vi "Vision Processing.vi"(4 "error in (no error)":errorcluster) -> ()   [LabVIEW 2019]
doc: "This VI runs in parallel to other tasks. It gets images from the camera, processes them for color or shape and uses commands or globals to affect the behavior of other subsystems."
uses:
  Framework/Robot Global Data.vi
  <vilib>/vision/NI_Vision_Development_Module.lvlib
panel:
  out "Results 2":T1(array[cluster]) {"Normalized Center"."x" format="%#_2g"; "Normalized Center"."y" format="%#_2g"; "Overall Score" format="%#_2g"; "Distance (ft)" format="%#_3g"; "Area Score" format="%#_2g"; "Moment Score" format="%#_2g"; "Aspect Score" format="%#_2g"}
  in  "Color Mode":u16(ring)=2 items=["RGB", "HSL", "HSV", "HSI"]
  out "Qualified 2":i32
  in  "LED Color Range":T2={"Hue"={92.46666717529297, 124.46666717529297}, "Sat"={154.82142857142856, 255.0}, "Val"={100.17857142857144, 251.32874298095703}} {"Hue" scale=0.0..255.0 scale format="%#_3g"}
  out "Results":T1(array[cluster]) {"Normalized Center"."x" format="%#_2g"; "Normalized Center"."y" format="%#_2g"; "Overall Score" format="%#_2g"; "Distance (ft)" format="%#_3g"; "Area Score" format="%#_2g"; "Moment Score" format="%#_2g"; "Aspect Score" format="%#_2g"}
  in  "Size Limit %":dbl=0.1 min=0.0 max=100.0 step=0.01 format="%#_13g"
  in  "Particle Count LImit":i32=5
  out "Qualified":i32
  out "Mask":T3(plugin-control)
  out "Original Image":T3(plugin-control)
  # "Scores"
  # "Scores"
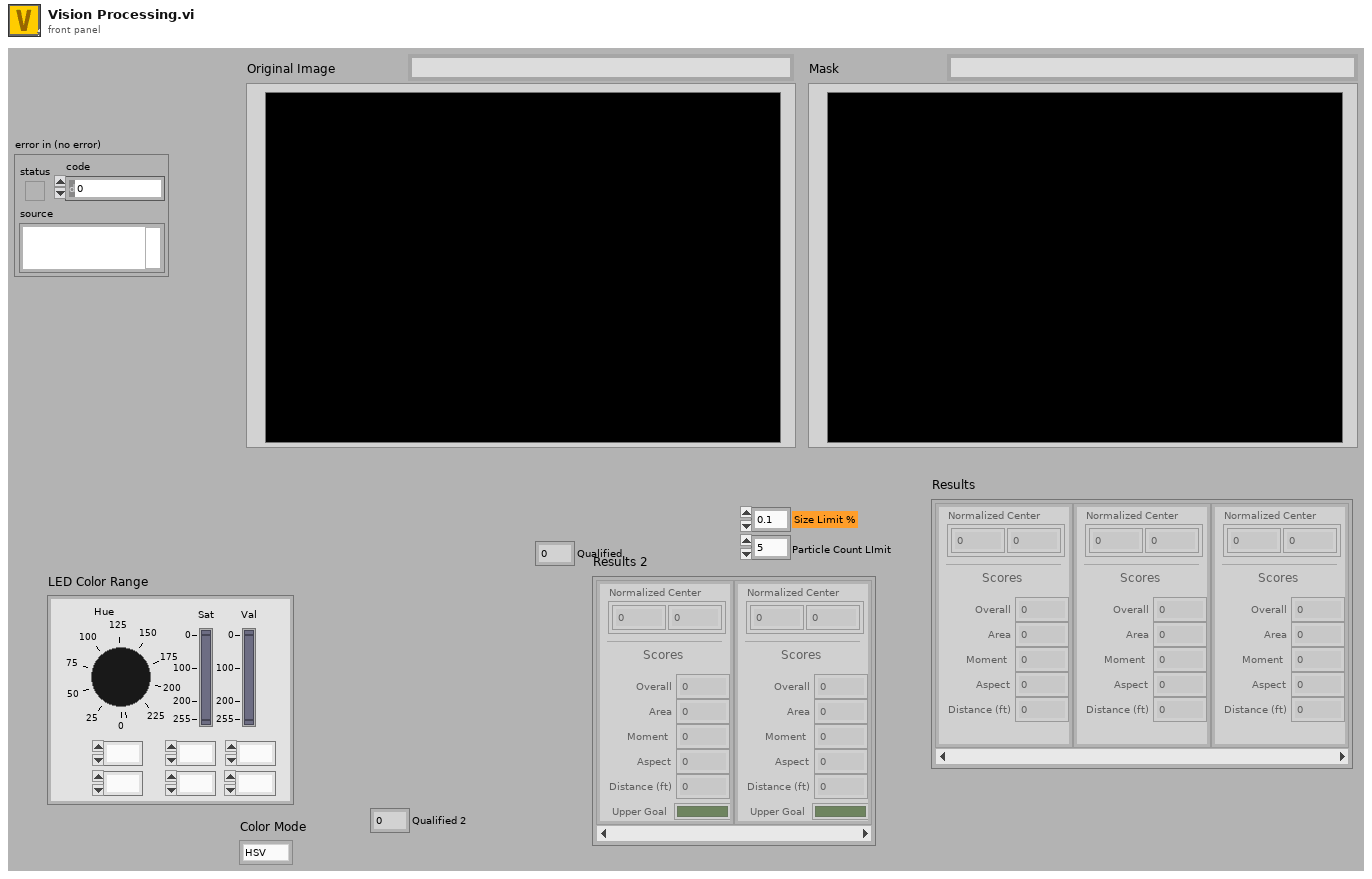
[diagram p1: front panel]
types:
  T1 = cluster{"diameter points":cluster{"first point":cluster{"x":dbl, "y":dbl}, "projected point":cluster{"x":dbl, "y":dbl}}, "Normalized Center":cluster{"x":dbl, "y":dbl}, "Overall Score":dbl, "Area Score":dbl, "Moment Score":dbl, "Aspect Score":dbl, "Distance (ft)":dbl, "Upper Goal":bool}[]
  T2 = cluster{"Hue":cluster{dbl, dbl}, "Sat":cluster{dbl, dbl}, "Val":cluster{dbl, dbl}}
  T3 = typedef "IMAQ Image.ctl" = refnum<image>
  T4 = typedef "Particle Parameters" = i32
  T5 = enum16{"Vision Off", "Ball Vision", "Feeder Station"}
  T6 = enum32{"AutoM", "Close", "Dilate", "Erode", "Gradient", "Gradient out", "Gradient in", "Hit miss", "Open", "PClose", "POpen", "Thick", "Thin"}
  T7 = typedef "Target Fields.ctl" = cluster{"diameter points":cluster{"first point":cluster{"x":dbl, "y":dbl}, "projected point":cluster{"x":dbl, "y":dbl}}, "normalized center":cluster{"x":dbl, "y":dbl}, "Overall Score":dbl, "Area Score":dbl, "Moment Score":dbl, "Aspect Score":dbl, "Distance (ft)":dbl, "Upper Goal":bool}
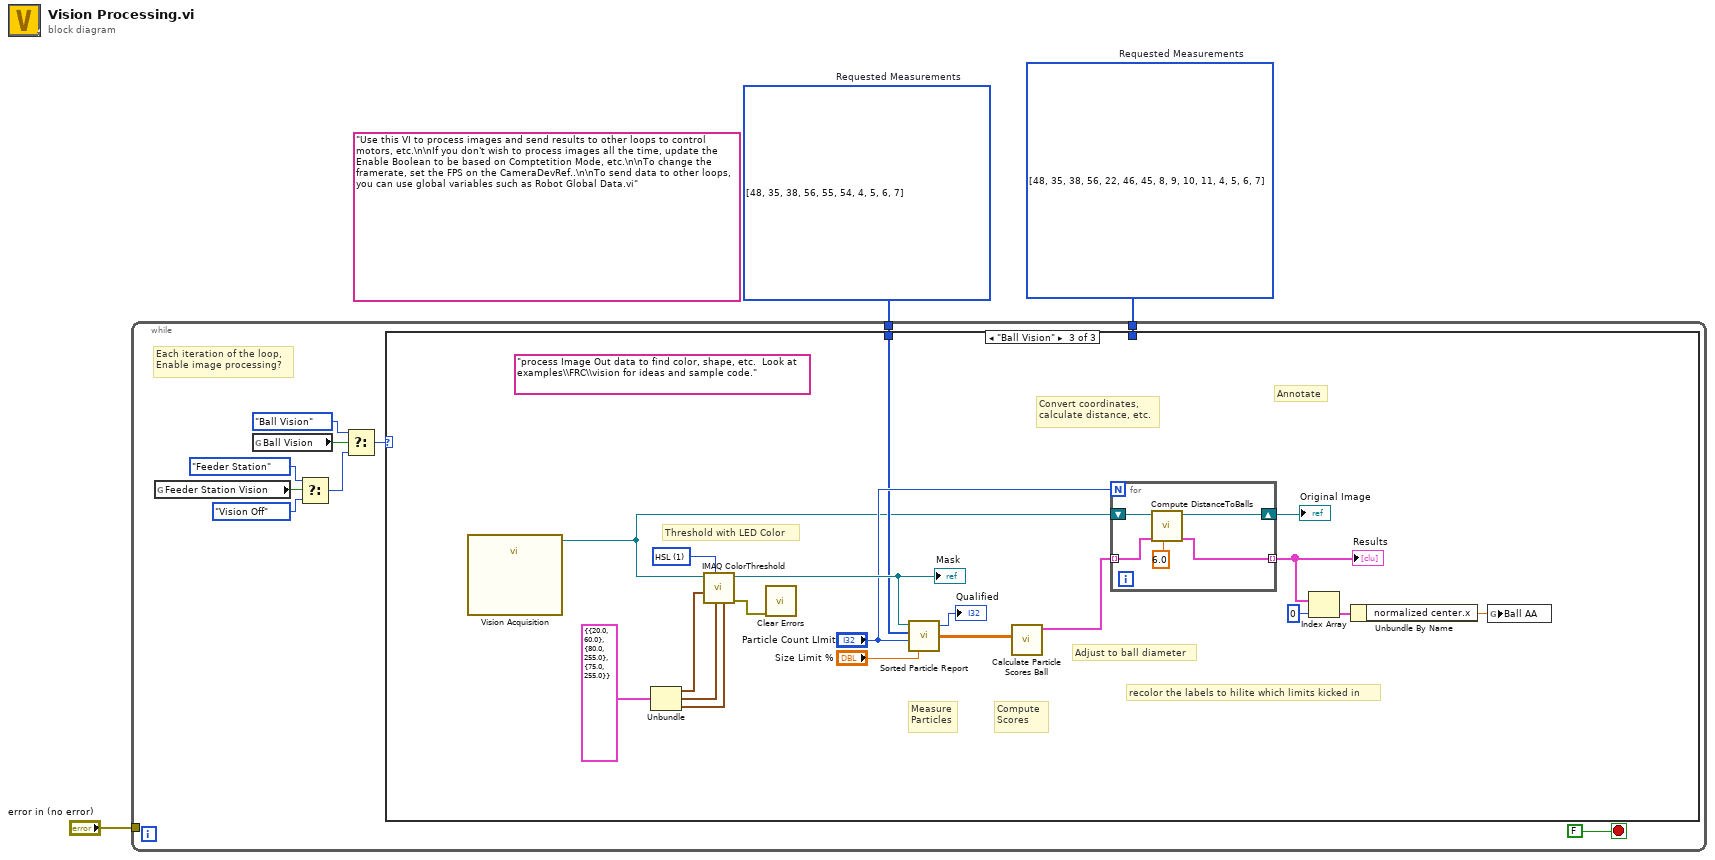
[diagram p0: block diagram]
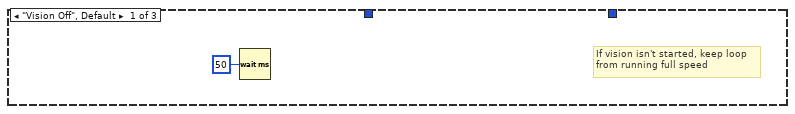
[diagram p2: hidden frame]
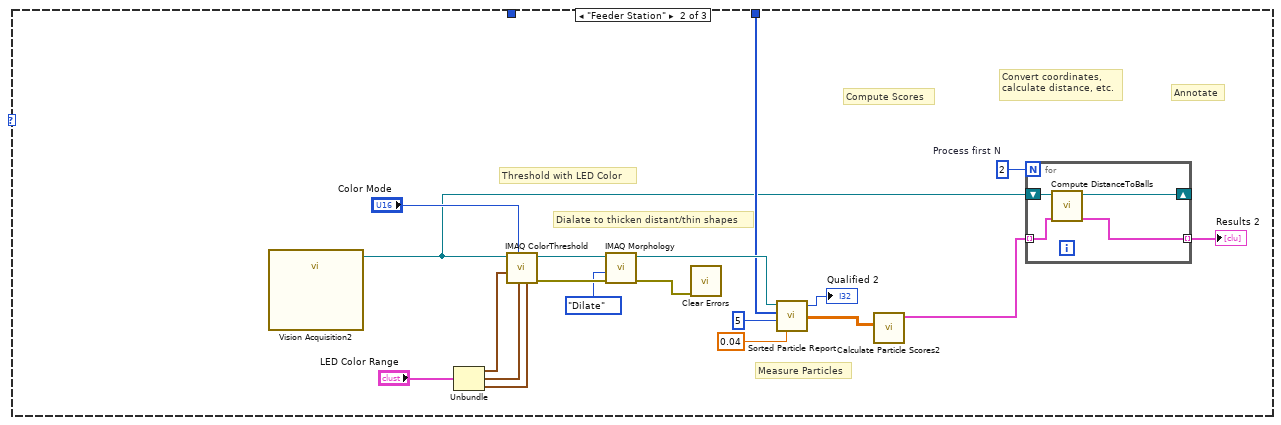
[diagram p3: hidden frame]
diagram:
  w1 = T4[] [48, 35, 38, 56, 22, 46, 45, 8, 9, 10, 11, 4, 5, 6, 7] items=["Center of Mass X", "Center of Mass Y", "First Pixel X", "First Pixel Y", "Bounding Rect Left", "Bounding Rect Top", "Bounding Rect Right", "Bounding Rect Bottom", "Max Feret Diameter Start X", "Max Feret Diameter Start Y", "Max Feret Diameter End X", "Max Feret Diameter End Y", "Max Horiz. Segment Length Left", "Max Horiz. Segment Length Right", "Max Horiz. Segment Length Row", "-", "Bounding Rect Width", "Bounding Rect Height", "Bounding Rect Diagonal", "Perimeter", "Convex Hull Perimeter", "Holes' Perimeter", "Max Feret Diameter", "Equivalent Ellipse Major Axis", "Equivalent Ellipse Minor Axis", "Equivalent Ellipse Minor Axis (Feret)", "Equivalent Rect Long Side", "Equivalent Rect Short Side", "Equivalent Rect Diagonal", "Equivalent Rect Short Side (Feret)", "Average Horiz. Segment Length", "Average Vert. Segment Length", "Hydraulic Radius", "Waddel Disk Diameter", "-", "Area", "Holes' Area", "Particle & Holes' Area", "Convex Hull Area", "Image Area", "-", "Number of Holes", "Number of Horiz. Segments", "Number of Vert. Segments", "-", "Orientation", "Max Feret Diameter Orientation", "-", "% Area/Image Area", "% Area/(Particle & Holes' Area)", "Ratio of Equivalent Ellipse Axes", "Ratio of Equivalent Rect Sides", "-", "Elongation Factor", "Compactness Factor", "Heywood Circularity Factor", "Type Factor", "-", "Sum X", "Sum Y", "Sum XX", "Sum XY", "Sum YY", "Sum XXX", "Sum XXY", "Sum XYY", "Sum YYY", "-", "Moment of Inertia XX", "Moment of Inertia XY", "Moment of Inertia YY", "Moment of Inertia XXX", "Moment of Inertia XXY", "Moment of Inertia XYY", "Moment of Inertia YYY", "Norm. Moment of Inertia XX", "Norm. Moment of Inertia XY", "Norm. Moment of Inertia YY", "Norm. Moment of Inertia XXX", "Norm. Moment of Inertia XXY", "Norm. Moment of Inertia XYY", "Norm. Moment of Inertia YYY", "Hu Moment 1", "Hu Moment 2", "Hu Moment 3", "Hu Moment 4", "Hu Moment 5", "Hu Moment 6", "Hu Moment 7"]  # Requested Measurements
  w2 = T4[] [48, 35, 38, 56, 55, 54, 4, 5, 6, 7] items=["Center of Mass X", "Center of Mass Y", "First Pixel X", "First Pixel Y", "Bounding Rect Left", "Bounding Rect Top", "Bounding Rect Right", "Bounding Rect Bottom", "Max Feret Diameter Start X", "Max Feret Diameter Start Y", "Max Feret Diameter End X", "Max Feret Diameter End Y", "Max Horiz. Segment Length Left", "Max Horiz. Segment Length Right", "Max Horiz. Segment Length Row", "-", "Bounding Rect Width", "Bounding Rect Height", "Bounding Rect Diagonal", "Perimeter", "Convex Hull Perimeter", "Holes' Perimeter", "Max Feret Diameter", "Equivalent Ellipse Major Axis", "Equivalent Ellipse Minor Axis", "Equivalent Ellipse Minor Axis (Feret)", "Equivalent Rect Long Side", "Equivalent Rect Short Side", "Equivalent Rect Diagonal", "Equivalent Rect Short Side (Feret)", "Average Horiz. Segment Length", "Average Vert. Segment Length", "Hydraulic Radius", "Waddel Disk Diameter", "-", "Area", "Holes' Area", "Particle & Holes' Area", "Convex Hull Area", "Image Area", "-", "Number of Holes", "Number of Horiz. Segments", "Number of Vert. Segments", "-", "Orientation", "Max Feret Diameter Orientation", "-", "% Area/Image Area", "% Area/(Particle & Holes' Area)", "Ratio of Equivalent Ellipse Axes", "Ratio of Equivalent Rect Sides", "-", "Elongation Factor", "Compactness Factor", "Heywood Circularity Factor", "Type Factor", "-", "Sum X", "Sum Y", "Sum XX", "Sum XY", "Sum YY", "Sum XXX", "Sum XXY", "Sum XYY", "Sum YYY", "-", "Moment of Inertia XX", "Moment of Inertia XY", "Moment of Inertia YY", "Moment of Inertia XXX", "Moment of Inertia XXY", "Moment of Inertia XYY", "Moment of Inertia YYY", "Norm. Moment of Inertia XX", "Norm. Moment of Inertia XY", "Norm. Moment of Inertia YY", "Norm. Moment of Inertia XXX", "Norm. Moment of Inertia XXY", "Norm. Moment of Inertia XYY", "Norm. Moment of Inertia YYY", "Hu Moment 1", "Hu Moment 2", "Hu Moment 3", "Hu Moment 4", "Hu Moment 5", "Hu Moment 6", "Hu Moment 7"]  # Requested Measurements
  (unwired) "Use this VI to process images and send results to other loops to control motors, etc.\n\nIf you don't wish to process images all the time, update the Enable Boolean to be based on Comptetition Mode, etc.\n\nTo change the framerate, set the FPS on the CameraDevRef..\n\nTo send data to other loops, you can use global variables such as Robot Global Data.vi"
  n1 = while {
    tunnel: "error in (no error)" -> [_]
    tunnel: w2 -> [w12]
    tunnel: w1 -> [w4]
    stop <- FALSE stop-if-true
    # "Each iteration of the loop,\nEnable image processing?"
    n2 = global read "Robot Global Data.vi" "Feeder Station Vision"() -> (w8:bool)
    n3 = global read "Robot Global Data.vi" "Ball Vision"() -> (w10:bool)
    n4 = Select(t=T5."Feeder Station", s=w8, f=T5."Vision Off") -> (s? t:f=w9:T5)
    n5 = Select(t=T5."Ball Vision", s=w10, f=w9) -> (s? t:f=w11:T5)
    n6 = case shown="\"Ball Vision\"" w11 {
      tunnel: w12 -> [_ _ w46]
      tunnel: w4 -> [_ w16 _]
      frame "Vision Off", Default {
        # "If vision isn't started, keep loop\nfrom running full speed"
        n7 = Wait (ms)(milliseconds to wait=u32 50) -> ()  [unwired: 1 out]
      }
      frame "Feeder Station" {
        w18 = 2  # Process first N
        # "Dialate to thicken distant/thin shapes"
        # "Measure Particles"
        # "Convert coordinates,\ncalculate distance, etc."
        # "Annotate"
        # "Compute Scores"
        # "Threshold with LED Color"
        n8 = call "Vision Acquisition2"() -> ("Image Out"=w15:T3)  [unwired: 25 in, 2 out]
        n9 = Unbundle("LED Color Range") -> ("Hue"=w19:cluster{dbl, dbl}, "Sat"=w20:cluster{dbl, dbl}, "Val"=w21:cluster{dbl, dbl})
        n10 = call "IMAQ ColorThreshold"("Blue or Luma or Val or Inten Range"=w21, "Green or Sat Range"=w20, "Color Mode"="Color Mode", "Red or Hue Range"=w19, "Image Src"=w15) -> ("error out"=w28:errorcluster, "Image Dst Out"=w27:T3)  [unwired: 5 in]
        n11 = call "IMAQ Morphology"("error in (no error)"=w28, "Operation"=T6."Dilate", "Image Src"=w27) -> ("error out"=w29:errorcluster, "Image Dst Out"=w32:T3)  [unwired: 7 in]
        n12 = call <vilib>:"Clear Errors.vi"("error in (no error)"=w29) -> ()  [unwired: 5 in, 2 out]
        n13 = call "Sorted Particle Report.vi"("Min Area Size %"=0.04 ("Size Limit % 2"), "Particle Count Limit"=5 ("Particle Count"), "Pixel Measurements"=w16, "Image in"=w32) -> ("Sorted Data"=w30:dbl[][], "Particles"=→"Qualified 2":i32)  [unwired: 1 out]
        n14 = call "Calculate Particle Scores2.vi"("Sorted Data"=w30) -> ("Scores"=w31:T7[])  [unwired: 10 in]
        n15 = for {
          N: w18 -> [_]
          tunnel: w31 -> [w35] mode=indexing
          shift-right: [w34] -> _
          shift-left: w15 -> [w37]
          tunnel: [w36] -> w33 mode=indexing
          n16 = call "Compute DistanceToBalls.vi"("results"=w35, "Image Src"=w37) -> ("results out"=w36:T7, "Image Dst Out"=w34:T3)  [unwired: 8 in]
        }
        "Results 2" <- w33
      }
      frame "Ball Vision" {
        w45 = u16 1 items=["RGB", "HSL", "HSV", "HSI"] ("Color Mode")
        (unwired) "process Image Out data to find color, shape, etc.  Look at examples\\FRC\\vision for ideas and sample code."
        # "recolor the labels to hilite which limits kicked in"
        # "Adjust to ball diameter"
        # "Measure\nParticles"
        # "Convert coordinates,\ncalculate distance, etc."
        # "Annotate"
        # "Compute\nScores"
        # "Threshold with LED Color"
        n17 = call "Vision Acquisition"() -> ("Image Out"=w40:T3)  [unwired: 25 in, 2 out]
        n18 = Unbundle(T2 {"Hue"={20.0, 60.0}, "Sat"={80.0, 255.0}, "Val"={75.0, 255.0}} ("cluster")) -> ("Hue"=w56:cluster{dbl, dbl}, "Sat"=w55:cluster{dbl, dbl}, "Val"=w54:cluster{dbl, dbl})
        n19 = call "IMAQ ColorThreshold"("Blue or Luma or Val or Inten Range"=w54, "Green or Sat Range"=w55, "Color Mode"=w45, "Red or Hue Range"=w56, "Image Src"=w40) -> ("error out"=w50:errorcluster, "Image Dst Out"=w51:T3)  [unwired: 5 in]
        "Mask" <- w51
        n20 = call <vilib>:"Clear Errors.vi"("error in (no error)"=w50) -> ()  [unwired: 5 in, 2 out]
        n21 = call "Sorted Particle Report.vi"("Min Area Size %"="Size Limit %", "Particle Count Limit"="Particle Count LImit", "Pixel Measurements"=w46, "Image in"=w51) -> ("Sorted Data"=w49:dbl[][], "Particles"=→"Qualified":i32)  [unwired: 1 out]
        n22 = call "Calculate Particle Scores Ball.vi"("Sorted Data"=w49) -> ("Scores"=w48:T7[])  [unwired: 10 in]
        n23 = for {
          N: "Particle Count LImit" -> [_]
          tunnel: w48 -> [w61] mode=indexing
          shift-right: [w57] -> w39
          shift-left: w40 -> [w59]
          tunnel: [w60] -> w43 mode=indexing
          n24 = call "Compute DistanceToBalls.vi"("Target Width (in)"=6.0, "results"=w61, "Image Src"=w59) -> ("results out"=w60:T7, "Image Dst Out"=w57:T3)  [unwired: 7 in]
        }
        "Original Image" <- w39
        "Results" <- w43
        n25 = Index Array(array=w43, index=0) -> (element=w41:T7)
        n26 = Unbundle By Name(w41) -> ("normalized center.x"=w38:dbl)
        n27 = global write "Robot Global Data.vi" "Ball AA"(w38) -> ()
      }
    }
  }
